vi "Locate Baseplate.vi"() -> ()   [LabVIEW 2016]
uses:
  Classes/Workspace/Workspace.ctl
  Classes/Workspace/Carrier Tray/Assembly Tray.lvclass
  Classes/Workspace/Component/Component Tray.lvclass
  Classes/Workspace/Pick Up Tool Area/Pick Up Tool.lvclass
  Classes/Controller/Controller.lvclass
  Classes/Workspace/Fixture.lvclass
panel:
  out "Workspace":T1
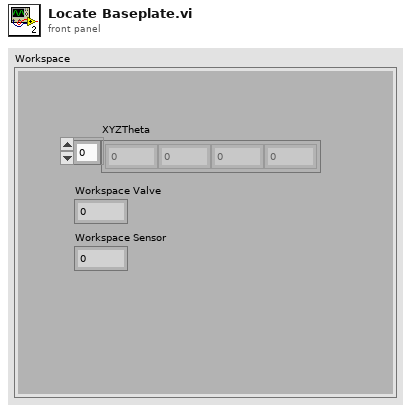
[diagram p1: front panel]
types:
  T1 = typedef "Fixture.lvclass/Workspace.ctl" = cluster{"XYZTheta":dbl[], "Workspace Valve":i32, "Workspace Sensor":i32}
  T2 = typedef "Controller.lvclass/Controllers.ctl" = cluster{"I-O.lvclass":refnum<class "I-O.lvclass">, "Motion.lvclass":refnum<class "Motion.lvclass">, "Dispenser.lvclass":refnum<class "Dispenser.lvclass">}
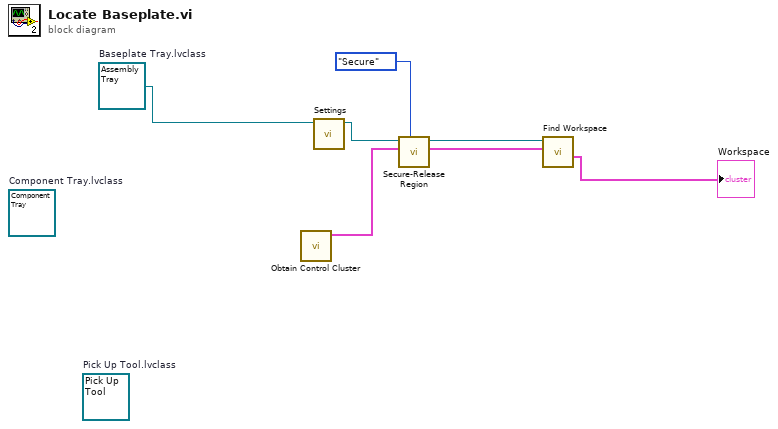
[diagram p0: block diagram]
diagram:
  (unwired) refnum<class "Pick Up Tool.lvclass"> refnum  # Pick Up Tool.lvclass
  (unwired) refnum<class "Component Tray.lvclass"> refnum  # Component Tray.lvclass
  w1 = refnum<class "Assembly Tray.lvclass"> refnum  # Baseplate Tray.lvclass
  n1 = call "Obtain Control Cluster.vi"() -> ("Control Out"=w4:T2)  [unwired: 11 in]
  n2 = call-dynamic "Settings.vi"("Baseplate Tray In"=w1) -> ("Baseplate Tray Out"=w7:refnum<class "Assembly Tray.lvclass">)  [unwired: 9 in, 1 out]
  n3 = call-dynamic "Secure-Release Region.vi"("Action"=enum16{"Secure", "Release"}."Secure", "Control In"=w4, "Baseplate Tray in"=w7) -> ("Control Out"=w3:T2, "Baseplate Tray out"=w6:refnum<class "Assembly Tray.lvclass">)  [unwired: 6 in, 1 out]
  n4 = call-dynamic "Find Workspace.vi"("Control In"=w3, "Baseplate Tray in"=w6) -> ("Workspace"=→"Workspace":T1)  [unwired: 6 in, 3 out]
